vi "Graph settings.vi"(11 "Settings in":T1={"Graph type"=1, "Scale"=1.0, "Offset"=0.0, "Automatic"=""} {"Graph type" items=["Mean(Y)", "Mean(X)"]}) -> (3 "Settings out":T1={"Graph type"=1, "Scale"=1.0, "Offset"=0.0, "Automatic"=""} {"Graph type" items=["Mean(Y)", "Mean(X)"]})   [LabVIEW 2018]
panel:
  in  "Cancel Button":bool
  in  "OK Button":bool
  in  "Tab Control":enum32{"Plot properties", "Scaling and units"}(tab)
  in  "Graph type":u16(ring)=1 items=["Mean(Y)", "Mean(X)"]
  in  "Automatic":string(combo)
  in  "Scale":dbl=1.0
  in  "Offset":dbl
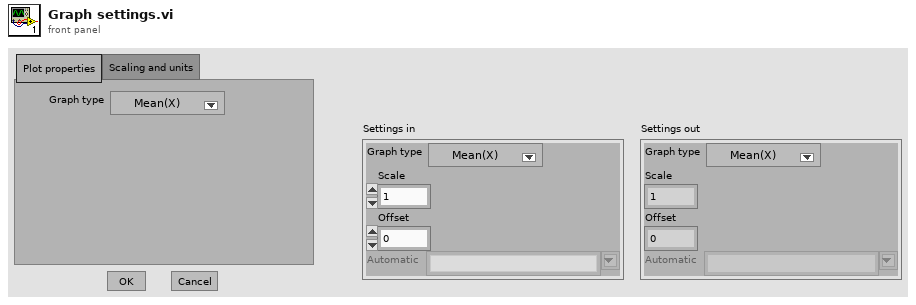
[diagram p1: front panel]
types:
  T1 = cluster{"Graph type":u16, "Scale":dbl, "Offset":dbl, "Automatic":string}
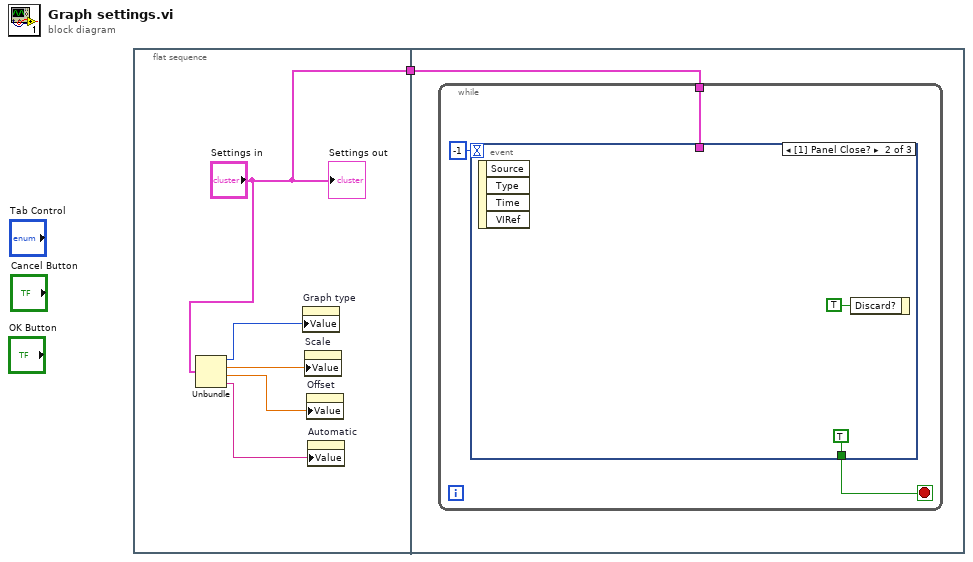
[diagram p0: block diagram]
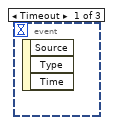
[diagram p2: hidden frame]
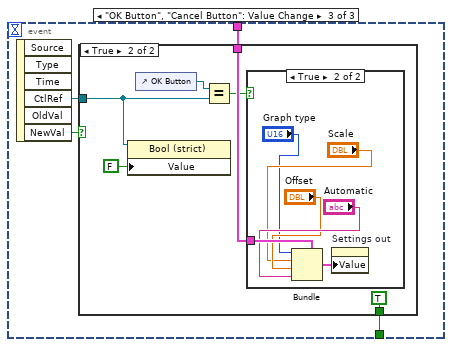
[diagram p3: hidden frame]
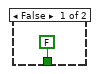
[diagram p4: hidden frame]
diagram:
  n1 = flat-sequence {
    tunnel: ["Settings in"] -> w1
    tunnel: w1 -> [w7]
    frame #0 {
      n2 = Unbundle("Settings in") -> ("Graph type"=w5:u16, "Scale"=w4:dbl, "Offset"=w3:dbl, "Automatic"=w2:string)
      n3 = property on="Graph type" class="Ring (strict)"("Value"=w5) -> ()  [unwired: 2 in, 2 out]
      n4 = property on="Scale" class="DigNum (strict)"("Value"=w4) -> ()  [unwired: 2 in, 2 out]
      n5 = property on="Offset" class="DigNum (strict)"("Value"=w3) -> ()  [unwired: 2 in, 2 out]
      n6 = property on="Automatic" class="CmbBox"("Value"=w2) -> ()  [unwired: 2 in, 2 out]
      "Settings out" <- "Settings in"
    }
    frame #1 {
      n7 = while {
        tunnel: w7 -> [w8]
        stop <- w9 stop-if-true
        n8 = event shown="[1] Panel Close?" {
          selector: _ -> [_ _ _]
          dyn-events: _ -> [_ _ _]
          timeout: -1 -> [_ _ _]
          tunnel: [_ TRUE w14] -> w9
          tunnel: w8 -> [_ _ w13]
          event Timeout {
            n9 = event-data() -> ()  [unwired: 1 in, 3 out]
          }
          event Panel Close? {
            n10 = event-data() -> ()  [unwired: 1 in, 4 out]
            n11 = event-data("Discard?"=TRUE) -> ()  [unwired: 1 in, 1 out]
          }
          event "OK Button", "Cancel Button": Value Change {
            n12 = event-data() -> ("CtlRef"=w15:refnum<vi>, "NewVal"=w16:bool)  [unwired: 1 in, 4 out]
            n13 = case shown="True" w16 {
              tunnel: w15 -> [_ w19]
              tunnel: [FALSE TRUE] -> w14
              tunnel: w13 -> [_ w21]
              frame False {
              }
              frame True {
                n14 = property class="Bool (strict)"(reference=w19, "Value"=FALSE) -> ()  [unwired: 1 in, 2 out]
                n15 = control-ref of="OK Button"() -> (w23:refnum<vi>)
                n16 = Equal?(x=w23, y=w19) -> (x = y?=w20:bool)
                n17 = case shown="True" w20 {
                  tunnel: w21 -> [_ w28]
                  frame False {
                  }
                  frame True {
                    n18 = Bundle(cluster=w28, "Graph type"="Graph type", "Scale"="Scale", "Offset"="Offset", "Automatic"="Automatic") -> (w29:T1)
                    n19 = property on="Settings out" class="Clust (strict)"("Value"=w29) -> ()  [unwired: 2 in, 2 out]
                  }
                }
              }
            }
          }
        }
      }
    }
  }
